vi "XY Plot - Area Bounds--Const.vi"() -> (3 "Plot Area Bounds":T1)   [LabVIEW 2017, in "DTacq Plot Display Library.lvlib"]
uses:
  DTacq Plot Display Library.lvlib
  <vilib>/Utility/miscctls.llb/LVRectTypeDef.ctl
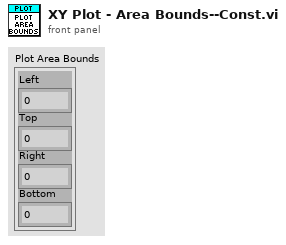
[diagram p1: front panel]
types:
  T1 = typedef "LVRectTypeDef.ctl" = cluster{"Left":i16, "Top":i16, "Right":i16, "Bottom":i16}
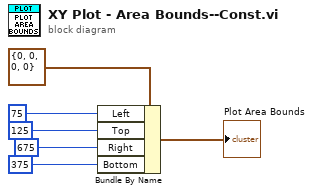
[diagram p0: block diagram]
diagram:
  n1 = Bundle By Name(cluster=T1 {"Left"=0, "Top"=0, "Right"=0, "Bottom"=0} ("Plot Area Bounds"), "Left"=i16 75, "Top"=i16 125, "Right"=i16 675, "Bottom"=i16 375) -> (→"Plot Area Bounds":T1)
